vi "tm422_firetriggerbutton.vi"() -> ()   [LabVIEW 2011]
panel:
  in  "Quit":bool
  in  "Snap":bool
  out "Image":u16[][](graph)
  out "Error Out":errorcluster
  # "This is a method to capture multiple single frames without reallocating the buffer."
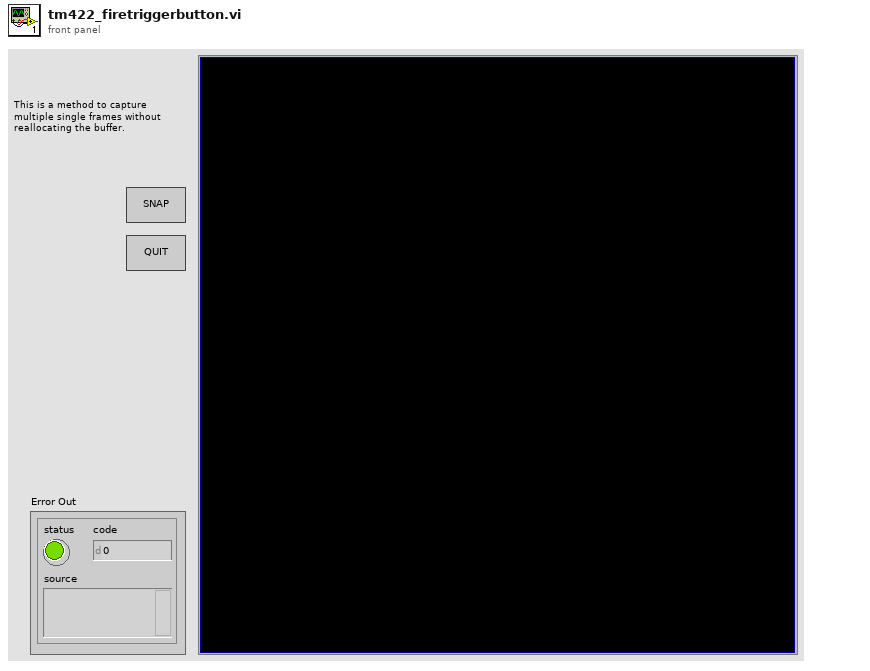
[diagram p1: front panel]
types:
  T1 = cluster{"Mode":u32, "Polarity":u32, "Times":u32, "Delay":dbl}
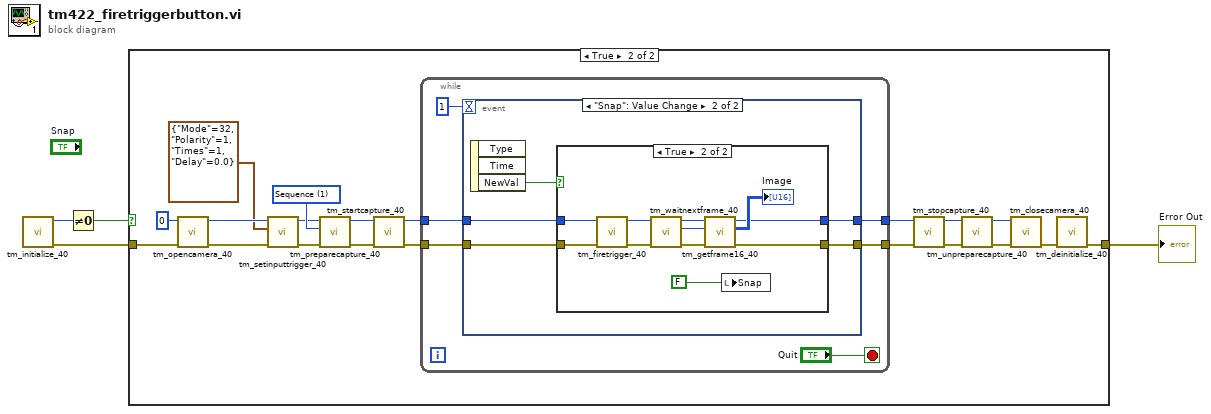
[diagram p0: block diagram]
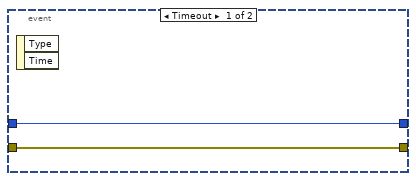
[diagram p3: hidden frame]
diagram:
  n1 = call <userlib>:"tm_initialize_40.vi"() -> ("error out"=w1:errorcluster, "Number Of Cameras"=w2:u32)  [unwired: 8 in, 2 out]
  n2 = Not Equal To 0?(x=w2) -> (x != 0?=w4:bool)
  n3 = case shown="True" w4 {
    tunnel: w1 -> [w5 w25]
    tunnel: [w5 w22] -> w3
    frame False {
    }
    frame True {
      w17 = 1 items=["Snap", "Sequence"] ("Capture mode")
      n4 = call <userlib>:"tm_opencamera_40.vi"("error in (no error)"=w25, "Camera Index"=u32 0) -> ("error out"=w9:errorcluster, "Handle out"=w10:u32)  [unwired: 7 in, 1 out]
      n5 = call <userlib>:"tm_setinputtrigger_40.vi"("error in (no error)"=w9, "Parameters"=T1 {"Mode"=32, "Polarity"=1, "Times"=1, "Delay"=0.0}, "Handle in"=w10) -> ("error out"=w7:errorcluster, "Handle out"=w8:u32)  [unwired: 7 in]
      n6 = call <userlib>:"tm_preparecapture_40.vi"("error in (no error)"=w7, "Capture mode"=w17, "Handle in"=w8) -> ("error out"=w14:errorcluster, "Handle out"=w13:u32)  [unwired: 5 in, 2 out]
      n7 = call <userlib>:"tm_startcapture_40.vi"("error in (no error)"=w14, "Handle in"=w13) -> ("error out"=w11:errorcluster, "Handle out"=w12:u32)  [unwired: 8 in]
      n8 = while {
        tunnel: w12 -> [w30]
        tunnel: w11 -> [w31]
        tunnel: [w29] -> w16
        tunnel: [w28] -> w15
        stop <- "Quit" stop-if-true
        n9 = event shown="[1] \"Snap\": Value Change" {
          selector: _ -> [_ _]
          dyn-events: _ -> [_ _]
          timeout: 1 -> [_ _]
          tunnel: w31 -> [w32 w38]
          tunnel: w30 -> [w33 w36]
          tunnel: [w33 w35] -> w29
          tunnel: [w32 w34] -> w28
          event Timeout {
            n10 = event-data() -> ()  [unwired: 1 in, 2 out]
          }
          event "Snap": Value Change {
            n11 = event-data() -> ("NewVal"=w37:bool)  [unwired: 1 in, 2 out]
            n12 = case shown="True" w37 {
              tunnel: w38 -> [w39 w45]
              tunnel: w36 -> [w40 w44]
              tunnel: [w40 w48] -> w35
              tunnel: [w39 w47] -> w34
              frame False {
              }
              frame True {
                n13 = call <userlib>:"tm_firetrigger_40.vi"("error in (no error)"=w45, "Handle in"=w44) -> ("error out"=w42:errorcluster, "Handle out"=w43:u32)  [unwired: 8 in]
                n14 = call <userlib>:"tm_waitnextframe_40.vi"("error in (no error)"=w42, "Handle in"=w43) -> ("error out"=w50:errorcluster, "Frame Index"=w41:i32, "Handle out"=w49:u32)  [unwired: 6 in, 1 out]
                n15 = call <userlib>:"tm_getframe16_40.vi"("error in (no error)"=w50, "Frame Index"=w41, "Handle in"=w49) -> ("error out"=w47:errorcluster, "Data"=→"Image":u16[][], "Handle out"=w48:u32)  [unwired: 5 in, 1 out]
                n16 = local write "Snap"(FALSE) -> ()
              }
            }
          }
        }
      }
      n17 = call <userlib>:"tm_stopcapture_40.vi"("error in (no error)"=w15, "Handle in"=w16) -> ("error out"=w18:errorcluster, "Handle out"=w19:u32)  [unwired: 8 in]
      n18 = call <userlib>:"tm_unpreparecapture_40.vi"("error in (no error)"=w18, "Handle in"=w19) -> ("error out"=w21:errorcluster, "Handle out"=w20:u32)  [unwired: 8 in]
      n19 = call <userlib>:"tm_closecamera_40.vi"("error in (no error)"=w21, "Handle in"=w20) -> ("error out"=w23:errorcluster)  [unwired: 9 in]
      n20 = call <userlib>:"tm_deinitialize_40.vi"("error in (no error)"=w23) -> ("error out"=w22:errorcluster)  [unwired: 10 in]
    }
  }
  "Error Out" <- w3
